vi "Proportional controller.vi"(9 "setpoint":dbl, 10 "measured":dbl, 11 "proportional control":dbl) -> (3 "output":dbl)   [LabVIEW 2014]
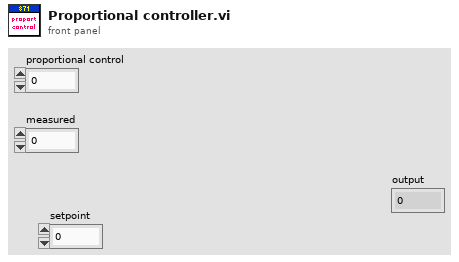
[diagram p1: front panel]
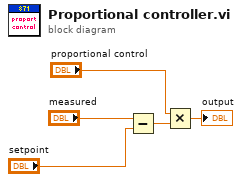
[diagram p0: block diagram]
diagram:
  n1 = Subtract(x="measured", y="setpoint") -> (x-y=w2:dbl)
  n2 = Multiply(x="proportional control", y=w2) -> (x*y=→"output":dbl)
